vi "get array from image file.vi"(8 "error in (no error)":errorcluster, 9 "ROI Descriptor Out":T1 {"Contours"."Type" items=["No Selection", "Point", "Line", "Rectangle", "Oval", "Polygon", "Freehand Region", "Annulus", "Unused2", "Unused3", "Broken Line", "Freehand Line", "Rotated Rectangle"]}, 10 "File Path":path, 11 "Autofocus in":refnum<class "Autofocus.lvclass">) -> (0 "error out":errorcluster, 1 "Image Source":T2(plugin-control), 2 "Array":dbl[][](array[numeric]), 3 "Autofocus out":refnum<class "Autofocus.lvclass">)   [LabVIEW 2012, in "Autofocus.lvclass"]
uses:
  Autofocus.lvclass
  Autofocus.lvclass/Autofocus.ctl
  <vilib>/vision/NI_Vision_Development_Module.lvlib
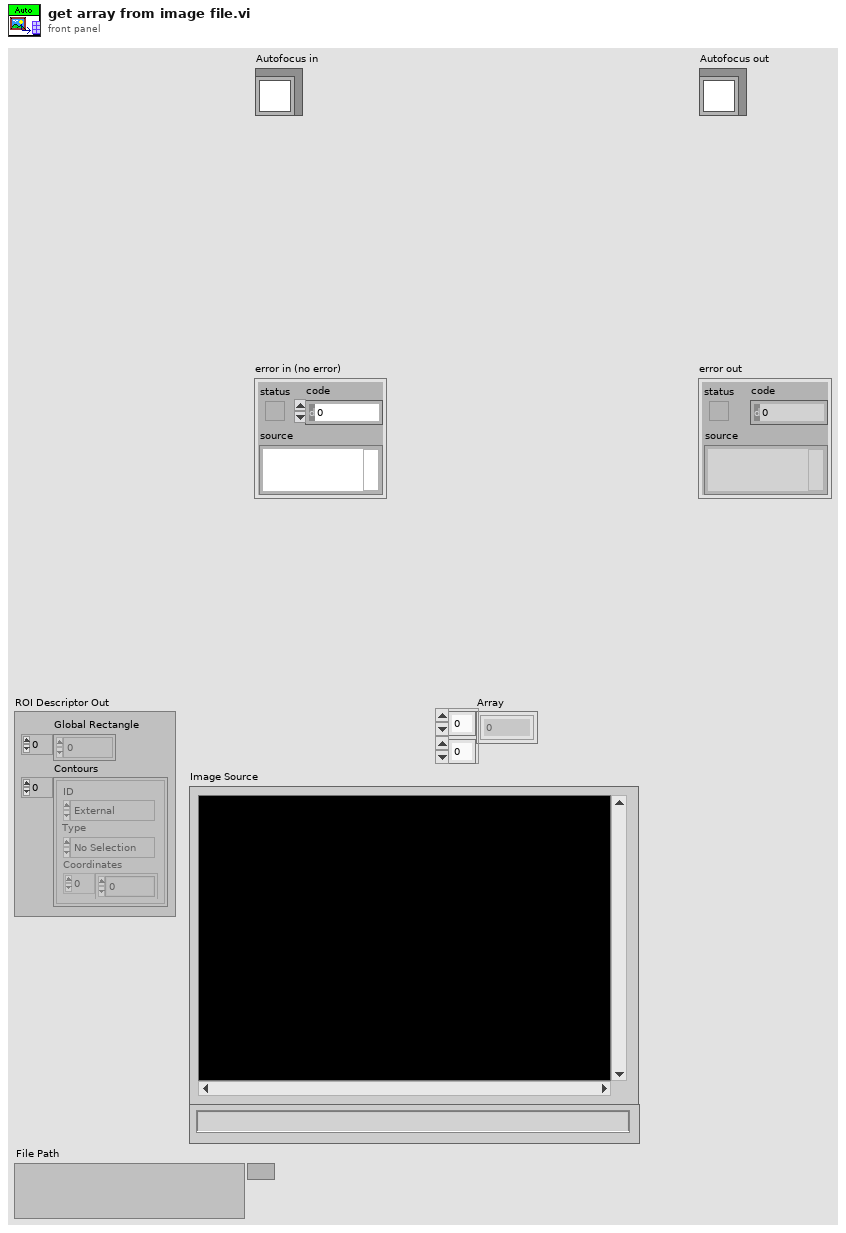
[diagram p1: front panel]
types:
  T1 = typedef "ROI Descriptor" = cluster{"Global Rectangle":i32[], "Contours":cluster{"ID":enum32{"External", "Internal"}, "Type":u32, "Coordinates":i32[]}[]}
  T2 = typedef "IMAQ Image.ctl" = refnum<image>
  T3 = typedef "Image Type" = u32
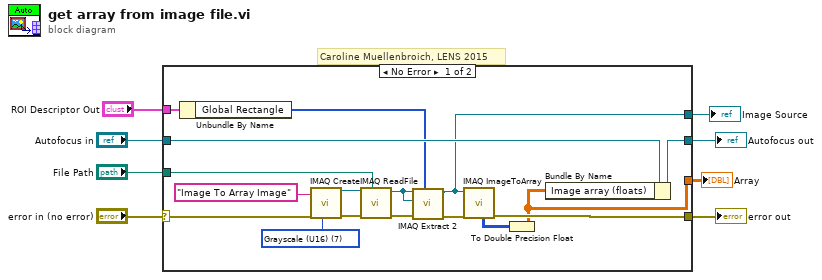
[diagram p0: block diagram]
diagram:
  # "Caroline Muellenbroich, LENS 2015"
  n1 = case shown="No Error" "error in (no error)" {
    selector: "error in (no error)" -> [w19 w27]
    tunnel: [w18 w27] -> w7
    tunnel: [w20 w26] -> w5
    tunnel: "Autofocus in" -> [w21 w26]
    tunnel: "File Path" -> [w17 _]
    tunnel: [w15 _] -> w3
    tunnel: [w12 _] -> w2
    tunnel: "ROI Descriptor Out" -> [w11 _]
    frame No Error {
      w22 = T3 7 items=["Grayscale (U8)", "Grayscale (I16)", "Grayscale (SGL)", "Complex (CSG)", "RGB (U32)", "HSL (U32)", "RGB (U64)", "Grayscale (U16)"] ("Image Type")
      n2 = Unbundle By Name(w11) -> ("Global Rectangle"=w10:i32[])
      n3 = call "IMAQ Create"("Image Name"="Image To Array Image", "Image Type"=w22, "error in (no error)"=w19) -> ("New Image"=w23:T2, "error out"=w24:errorcluster)  [unwired: 2 in]
      n4 = call "IMAQ ReadFile"("File Path"=w17, "error in (no error)"=w24, "Image"=w23) -> ("error out"=w14:errorcluster, "Image Out"=w9:T2)  [unwired: 4 in, 3 out]
      n5 = call "IMAQ Extract 2"("Optional Rectangle"=w10, "error in (no error)"=w14, "Image Dst"=w9, "Image Src"=w9) -> ("error out"=w13:errorcluster, "Image Dst Out"=w12:T2)  [unwired: 6 in]
      n6 = call "IMAQ ImageToArray"("error in (no error)"=w13, "Image"=w12) -> ("Image Pixels (U16)"=w16:u16[][], "error out"=w18:errorcluster)  [unwired: 2 in, 3 out]
      n7 = To Double Precision Float(number=w16) -> (double precision float=w15:dbl[][])
      n8 = Bundle By Name(cluster=w21, "Image array (floats)"=w15) -> (w20:refnum<class "Autofocus.lvclass">)
    }
    frame Error {
    }
  }
  "error out" <- w7
  "Autofocus out" <- w5
  "Array" <- w3
  "Image Source" <- w2
